vi "Teleop.vi"(10 "Match Info":T1={"Autonomous Elapsed Seconds"=0.0, "TeleOp Elapsed Seconds"=0.0, "Disabled Elapsed Seconds"=0.0, "Visited Autonomous"=FALSE, "Visited TeleOp"=FALSE, "Visited Disabled"=FALSE, "Autonomous Settings"={"Autonomous Style"=enum."Independent", "VI Refnum"=refnum}}, 11 "Call Context":T2) -> ()   [LabVIEW 2016]
doc: "This VI is called for each TeleOp packet received from the DS where the robot is not disabled. It is often used to read from the joysticks and update I/O or to update setpoints for timed control loops. It should complete and return within 20 milliseconds or it may miss DS packets."
uses:
  <vilib>/Rock Robotics/WPI/DriverStation/WPI_DriverStationDerivedRobotMode.ctl
  <vilib>/Rock Robotics/WPI/DriverStation/WPI_DriverStationMatch Info.ctl
  <vilib>/Rock Robotics/WPI/Solenoid/WPI_SolenoidValue.ctl
  <vilib>/Rock Robotics/WPI/Utilities/WPI_GetSetVariantRefNum.vi
  <vilib>/Rock Robotics/WPI/Joystick/WPI_JoystickArcadeMapping.vi
  <vilib>/Rock Robotics/Network Tables/NT Read Number.vi
  <vilib>/Rock Robotics/Network Tables/NT Read Boolean.vi
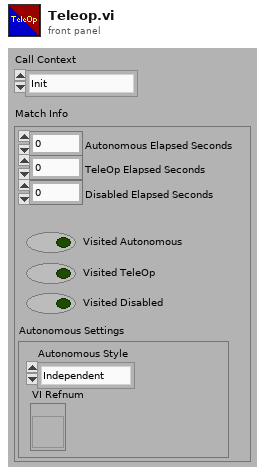
[diagram p1: front panel]
types:
  T1 = typedef "WPI_DriverStationMatch Info.ctl" = cluster{"Autonomous Elapsed Seconds":dbl, "TeleOp Elapsed Seconds":dbl, "Disabled Elapsed Seconds":dbl, "Visited Autonomous":bool, "Visited TeleOp":bool, "Visited Disabled":bool, "Autonomous Settings":cluster{"Autonomous Style":enum16{"Iterative", "Independent"}, "VI Refnum":refnum<vi>}}
  T2 = typedef "WPI_DriverStationDerivedRobotMode.ctl" = enum16{"Init", "Execute", "Stop"}
  T3 = typedef "WPI_SolenoidValue.ctl" = enum16{"Off", "On", "Forward", "Reverse"}
  T4 = typedef "WPI_JoystickDevRef.ctl" = cluster{"Device":T5}
  T5 = typedef "WPI_JoystickDeviceEnum.ctl" = enum16{"USB 0", "USB 1", "USB 2", "USB 3", "USB 4", "USB 5"}
  T6 = typedef "WPI_MotorControlDeviceRef.ctl" = cluster{"DeviceStatus":errorcluster, "Type":T7, "PWM":cluster{"PWM Channel":T8, "DeadBand":T9}, "CAN":cluster{"Device Number":u8, "SetOutput VI Ref":variant, "GetOutput VI Ref":variant, "Enable VI Ref":variant, "Disable VI Ref":variant, "Data":variant}, "Invert":bool}
  T7 = typedef "WPI_MotorControlType.ctl" = enum16{"PWM", "CAN"}
  T8 = typedef "FPGA_DIOPWMChannel.ctl" = enum8{"PWM 0", "PWM 1", "PWM 2", "PWM 3", "PWM 4", "PWM 5", "PWM 6", "PWM 7", "PWM 8", "PWM 9", "PWM MXP 0", "PWM MXP 1", "PWM MXP 2", "PWM MXP 3", "PWM MXP 4", "PWM MXP 5", "PWM MXP 6", "PWM MXP 7", "PWM MXP 8", "PWM MXP 9", "Invalid"}
  T9 = typedef "WPI_PWMDeadband.ctl" = cluster{"Name":string, "maxPositivePwm":i32, "minPositivePwm":i32, "centerPwm":i32, "maxNegativePwm":i32, "minNegativePwm":i32, "angularRange":u16}
  T10 = typedef "WPI_SolenoidDevRef.ctl" = cluster{"DevStatus":errorcluster, "Pneumatics Control Module":u8, "Forward Solenoid Channel":T11, "Reverse Solenoid Channel":T11}
  T11 = typedef "WPI_SolenoidChannel.ctl" = enum8{"Solenoid 0", "Solenoid 1", "Solenoid 2", "Solenoid 3", "Solenoid 4", "Solenoid 5", "Solenoid 6", "Solenoid 7", "Invalid"}
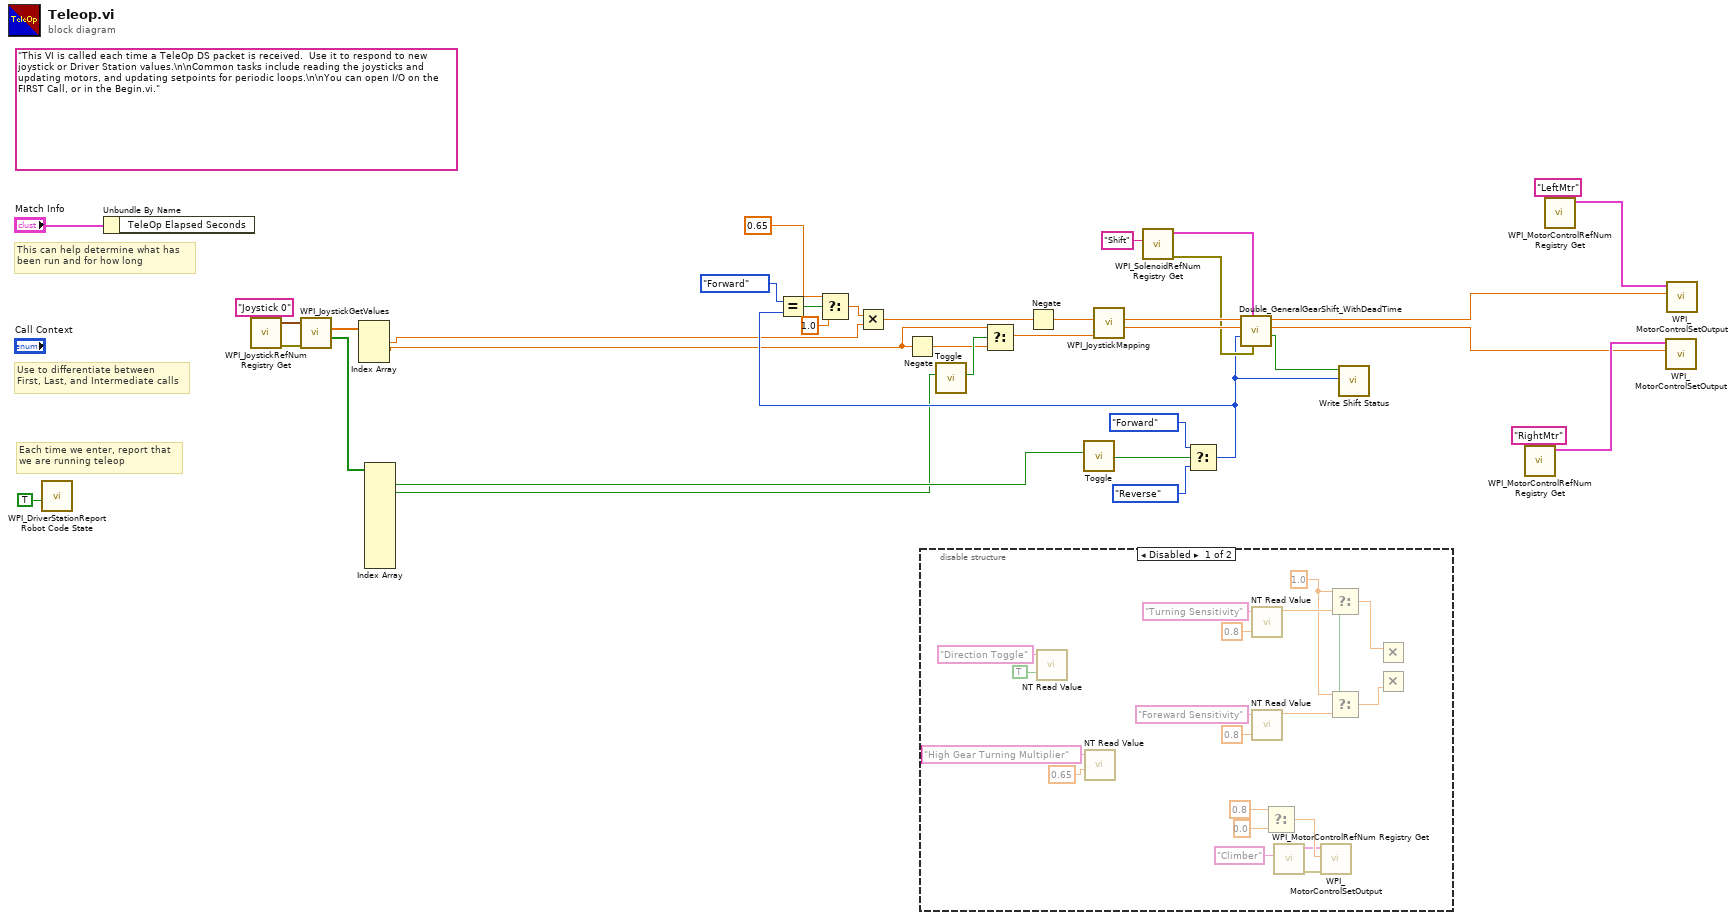
[diagram p0: block diagram]
diagram:
  (unwired) "This VI is called each time a TeleOp DS packet is received.  Use it to respond to new joystick or Driver Station values.\n\nCommon tasks include reading the joysticks and updating motors, and updating setpoints for periodic loops.\n\nYou can open I/O on the FIRST Call, or in the Begin.vi."
  # "Each time we enter, report that\nwe are running teleop"
  # "Use to differentiate between\nFirst, Last, and Intermediate calls"
  # "This can help determine what has\nbeen run and for how long"
  n1 = call <vilib>:"WPI_DriverStationReport Robot Code State.vi"("TeleOp"=TRUE ("Autonomous")) -> ()  [unwired: 10 in, 1 out]
  n2 = Unbundle By Name("Match Info") -> ()  [unwired: 1 out]
  n3 = call <vilib>:"WPI_JoystickRefNum Registry Get.vi"("refnum name"="Joystick 0") -> ("error out"=w31:errorcluster, "JoystickDevRef"=w34:T4)  [unwired: 1 in, 8 out]
  n4 = call <vilib>:"WPI_JoystickGetValues.vi"("error in (no error)"=w31, "JoystickDevRef"=w34) -> ("Buttons"=w32:bool[], "Axes"=w33:dbl[])  [unwired: 5 in, 3 out]
  n5 = Index Array(array=w33) -> (element #1=w4:dbl, element #2=w3:dbl)  [unwired: 3 in, 1 out]
  n6 = Index Array(array=w32) -> (element #1=w17:bool, element #2=w1:bool)  [unwired: 11 in, 9 out]
  n7 = Negate(x=w3) -> (-x=w29:dbl)
  n8 = disable-structure shown="Disabled" {
    frame Disabled {
      w49 = 1.0 ("t")
      n9 = call-poly <vilib>:"NT Read Value.vi"("Default Value"=TRUE, "Name"="Direction Toggle") -> ()  [unwired: 8 in, 2 out]
      n10 = call-poly <vilib>:"NT Read Value.vi"("Default Value"=0.65, "Name"="High Gear Turning Multiplier") -> ()  [unwired: 8 in, 2 out]
      n11 = call-poly <vilib>:"NT Read Value.vi"("Default Value"=0.8, "Name"="Turning Sensitivity") -> ("Numeric"=w51:dbl)  [unwired: 8 in, 1 out]
      n12 = call-poly <vilib>:"NT Read Value.vi"("Default Value"=0.8, "Name"="Foreward Sensitivity") -> ("Numeric"=w53:dbl)  [unwired: 8 in, 1 out]
      n13 = Select(t=0.8, f=0.0) -> (s? t:f=w44:dbl)  [unwired: 1 in]
      n14 = call <vilib>:"WPI_MotorControlRefNum Registry Get.vi"("refnum name"="Climber") -> ("error out"=w42:errorcluster, "MotorControlDevRef"=w43:T6)  [unwired: 9 in]
      n15 = call <vilib>:"WPI_MotorControlSetOutput.vi"("error in (no error)"=w42, "Output"=w44, "MotorControlDevRef"=w43) -> ()  [unwired: 6 in, 3 out]
      n16 = Select(t=w49, f=w53) -> (s=w48:bool, s? t:f=w52:dbl)
      n17 = Select(t=w49, s=w48, f=w51) -> (s? t:f=w50:dbl)
      n18 = Multiply(x=w50) -> (y=w55:dbl)  [unwired: 1 out]
      n19 = Multiply(y=w52) -> (x=w54:dbl)  [unwired: 1 out]
    }
    frame Enabled {
    }
  }
  n20 = call "Toggle.vi"("Input"=w1) -> ("Output"=w30:bool)  [unwired: 10 in]
  n21 = Select(t=w3, s=w30, f=w29) -> (s? t:f=w7:dbl)
  n22 = call "Toggle.vi"("Input"=w17) -> ("Output"=w20:bool)  [unwired: 10 in]
  n23 = call <vilib>:"WPI_SolenoidRefNum Registry Get.vi"("refnum name"="Shift") -> ("error out"=w14:errorcluster, "SolenoidDevRef"=w15:T10)  [unwired: 9 in]
  n24 = Select(t=WPI_SolenoidValue."Forward" ("Shift Value"), s=w20, f=WPI_SolenoidValue."Reverse" ("Shift Value")) -> (s? t:f=w10:T3)
  n25 = Equal?(x=WPI_SolenoidValue."Forward" ("Shift Value"), y=w10) -> (x = y?=w12:bool)
  n26 = Select(t=0.65, s=w12, f=1.0) -> (s? t:f=w8:dbl)
  n27 = Multiply(x=w8, y=w4) -> (x*y=w6:dbl)
  n28 = Negate(x=w6) -> (-x=w5:dbl)
  n29 = call-poly <vilib>:"WPI_JoystickMapping.vi"("Y axis value"=w7, "X axis value"=w5) -> ("Right Motor Value"=w23:dbl, "Left Motor Value"=w24:dbl)  [unwired: 8 in]
  n30 = call "Double_GeneralGearShift_WithDeadTime.vi"("error In"=w14, "ShifterRef"=w15, "Shift Value"=w10, "Right"=w23, "Left"=w24) -> ("Shifting"=w13:bool, "Right Output"=w21:dbl, "Left Output"=w22:dbl)  [unwired: 3 in, 1 out]
  n31 = call "Write Shift Status.vi"("Gear"=w10, "Output"=w13) -> ()  [unwired: 9 in, 1 out]
  n32 = call <vilib>:"WPI_MotorControlRefNum Registry Get.vi"("refnum name"="RightMtr") -> ("MotorControlDevRef"=w27:T6)  [unwired: 9 in, 1 out]
  n33 = call <vilib>:"WPI_MotorControlRefNum Registry Get.vi"("refnum name"="LeftMtr") -> ("MotorControlDevRef"=w28:T6)  [unwired: 9 in, 1 out]
  n34 = call <vilib>:"WPI_MotorControlSetOutput.vi"("Output"=w21, "MotorControlDevRef"=w27) -> ()  [unwired: 7 in, 3 out]
  n35 = call <vilib>:"WPI_MotorControlSetOutput.vi"("Output"=w22, "MotorControlDevRef"=w28) -> ()  [unwired: 7 in, 3 out]
